vi "BlinkM PlayLightScript.vi"(0 "Arduino Resource":T1={"VISA resource"="", "Board Type"=enum."Uno", "Connection Type"=enum."USB / Serial", "Bytes Per Packet (15)"=15}, 1 "BlinkM Script (User Script)":T3, 5 "Address (0)":u8, 7 "Number Of Repeats (0)":u8, 9 "Starting Script Line (0)":u8, 11 "error in":errorcluster) -> (4 "Arduino Resource":T1={"VISA resource"="", "Board Type"=enum."Uno", "Connection Type"=enum."USB / Serial", "Bytes Per Packet (15)"=15}, 15 "error out":errorcluster)   [LabVIEW 2015, in "LabVIEW Interface for Arduino.lvlib"]
doc: "Play light script stored on the BlinkM"
uses:
  <vilib>/LabVIEW Interface for Arduino/LabVIEW Interface for Arduino.lvlib
  <vilib>/LabVIEW Interface for Arduino/Type Defs/BlinkM Script.ctl
  <vilib>/LabVIEW Interface for Arduino/Type Defs/Arduino Resource.ctl
  <vilib>/LabVIEW Interface for Arduino/Type Defs/Board Type.ctl
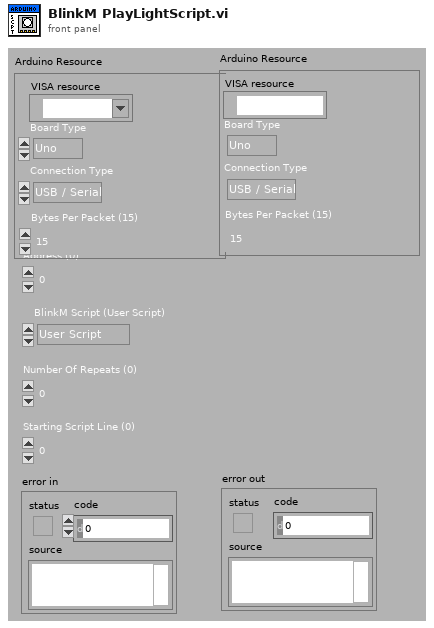
[diagram p1: front panel]
types:
  T1 = typedef "LabVIEW Interface for Arduino.lvlib/Arduino Resource.ctl" = cluster{"VISA resource":refnum<visa-resource-name>, "Board Type":T2, "Connection Type":enum8{"USB / Serial"}, "Bytes Per Packet (15)":u8}
  T2 = typedef "LabVIEW Interface for Arduino.lvlib/Board Type.ctl" = enum16{"Uno", "Dimuelanove w/Atmega 328", "Mega 2560"}
  T3 = typedef "LabVIEW Interface for Arduino.lvlib/BlinkM Script.ctl" = enum8{"User Script", "RGB", "White Flash", "Red Flash", "Green Flash", "Blue Flash", "Cyan Flash", "Magenta Flash", "Yellow Flash", "Black", "Hue Cycle", "Mood Light", "Virtual Candle", "Water Reflections", "Old Neon", "The Seasons", "Thunderstorm", "Stop Light", "Morse Code S.O.S"}
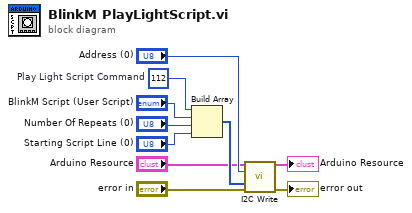
[diagram p0: block diagram]
diagram:
  w7 = u8 112  # Play Light Script Command
  n1 = Build Array(w7, "BlinkM Script (User Script)", "Number Of Repeats (0)", "Starting Script Line (0)") -> (w6:u8[])
  n2 = call <vilib>:"I2C Write.vi"("Arduino Resource"="Arduino Resource", "Address (0)"="Address (0)", "I2C Data Bytes"=w6, "error in"="error in") -> ("Arduino Resource"=→"Arduino Resource":T1, "error out"=→"error out":errorcluster)  [unwired: 10 in]
